vi "Log_Comando.vi"(0 "Porta":refnum<visa-resource-name>, 1 "Erro":bool, 2 "string do Comando":string, 3 "string da resposta":string, 4 "String":string, 5 "Erro de Resposta":bool, 6 "Erro Recebido":bool) -> ()   [LabVIEW 2018]
uses:
  Global_Telescopio.vi
panel:
  out "before substring":string
  out "Comando":string
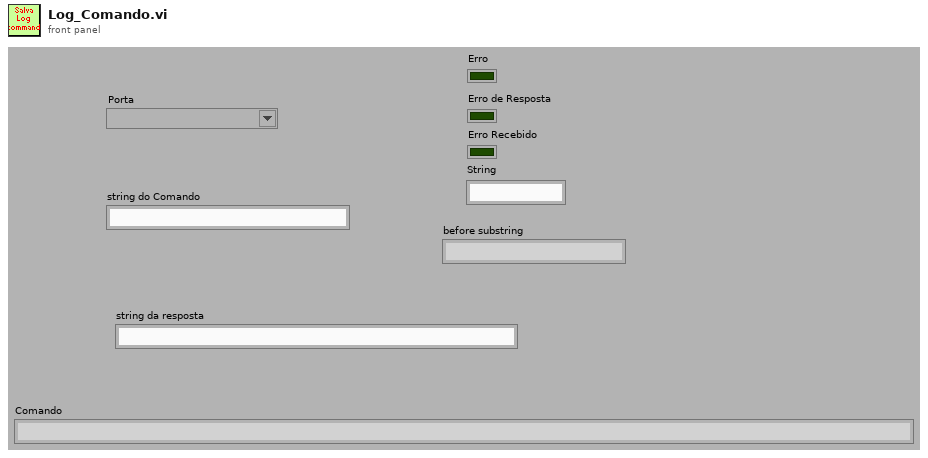
[diagram p1: front panel]
types:
  T1 = enum16{"open", "open or create", "create or replace", "create"}
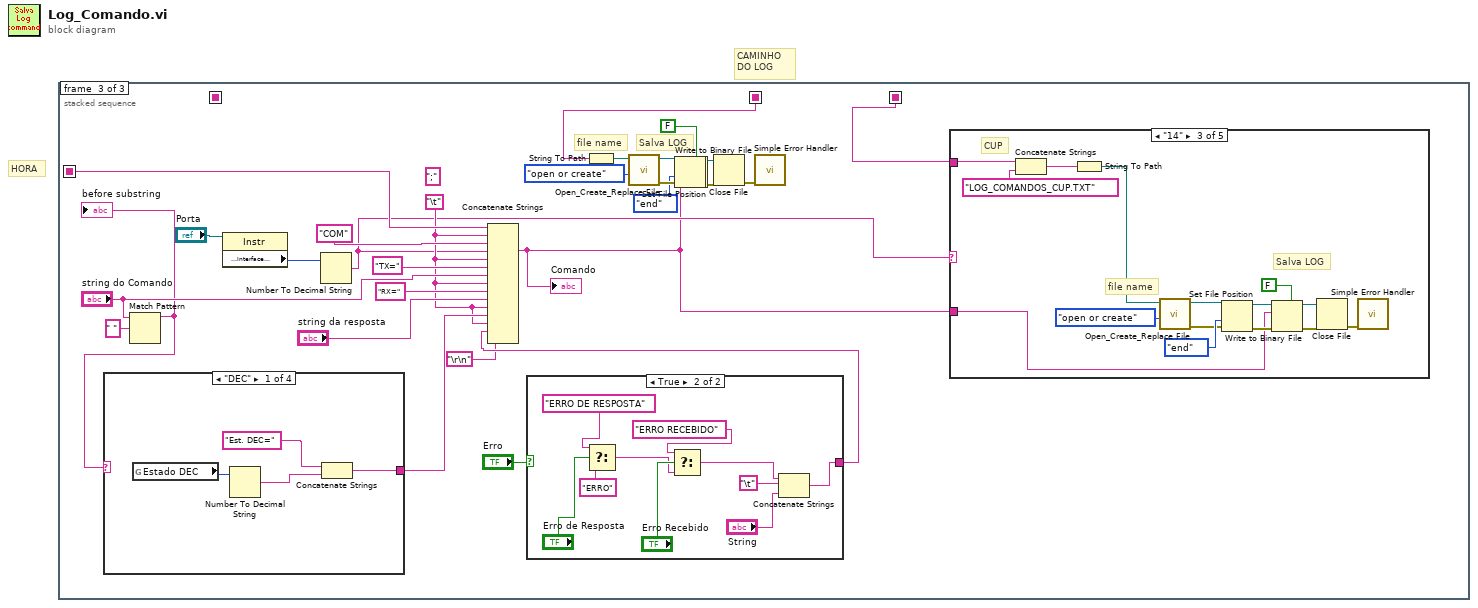
[diagram p0: block diagram]
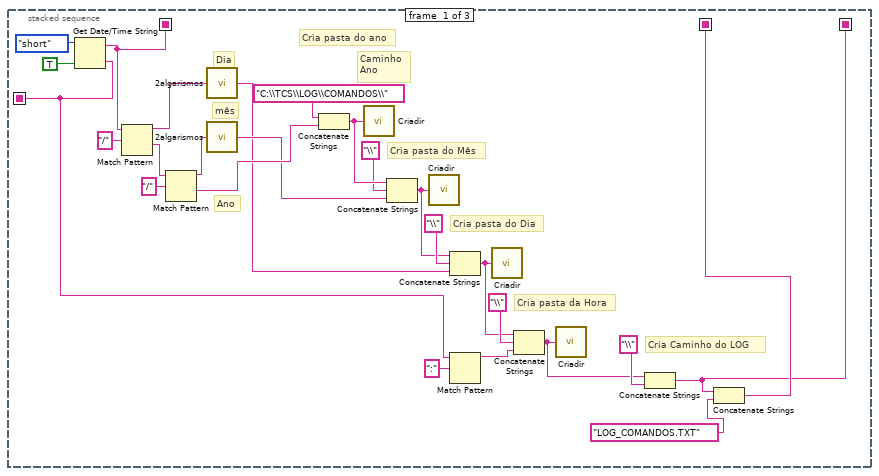
[diagram p2: hidden frame]
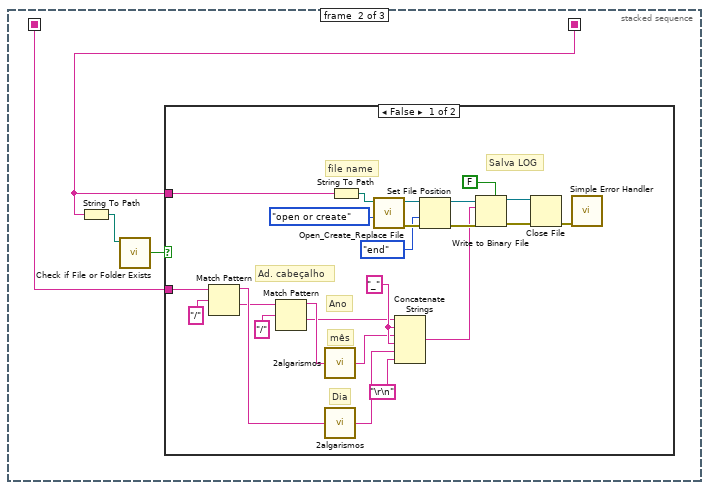
[diagram p3: hidden frame]
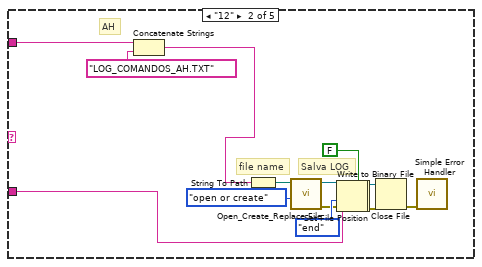
[diagram p6: hidden frame]
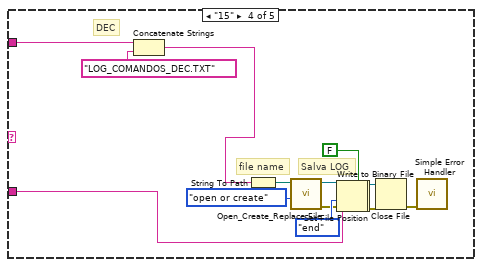
[diagram p7: hidden frame]
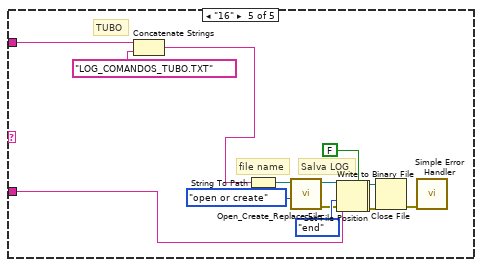
[diagram p8: hidden frame]
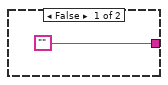
[diagram p9: hidden frame]
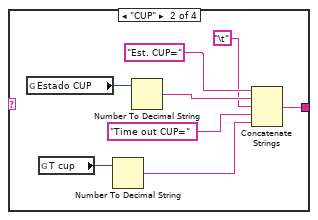
[diagram p10: hidden frame]
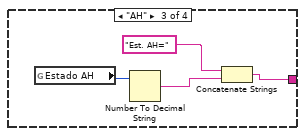
[diagram p11: hidden frame]
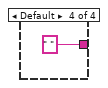
[diagram p12: hidden frame]
diagram:
  # "HORA"
  # "CAMINHO\nDO LOG"
  n1 = stacked-sequence {
    seq-local: [w2 _ _] -> [_ w29 w57]
    seq-local: [w7 _ _] -> [_ _ w81]
    seq-local: [w4 _ _] -> [_ w30 _]
    seq-local: [w1 _ _] -> [_ _ w55]
    frame #0 {
      # "Cria pasta da Hora"
      # "Cria Caminho do LOG"
      # "Cria pasta do Dia"
      # "Cria pasta do Mês"
      # "Caminho\nAno"
      # "Ano"
      # "mês"
      # "Dia"
      # "Cria pasta do ano"
      n2 = Get Date/Time String(date format (0)=enum16{"short", "long", "abbreviated"}."short", want seconds? (F)=TRUE) -> (date string=w4:string, time string=w7:string)  [unwired: 1 in]
      n3 = Match Pattern(string=w4, regular expression="/") -> (before substring=w23:string, after substring=w24:string)  [unwired: 1 in, 2 out]
      n4 = Match Pattern(string=w24, regular expression="/") -> (before substring=w22:string, after substring=w20:string)  [unwired: 1 in, 2 out]
      n5 = call "2algarismos.vi"("entrada"=w23) -> ("saida"=w14:string)
      n6 = call "2algarismos.vi"("entrada"=w22) -> ("saida"=w17:string)
      n7 = Concatenate Strings("C:\\TCS\\LOG\\COMANDOS\\" ("SOMENTE DIRETORIO"), w20) -> (w19:string)
      n8 = call "Criadir.vi"("SOMENTE DIRETORIO"=w19) -> ()  [unwired: 2 out]
      n9 = Concatenate Strings(w19, "\\" ("regular expression"), w17) -> (w15:string)
      n10 = call "Criadir.vi"("SOMENTE DIRETORIO"=w15) -> ()  [unwired: 2 out]
      n11 = Concatenate Strings(w15, "\\" ("regular expression"), w14) -> (w9:string)
      n12 = Match Pattern(string=w7, regular expression=":") -> (before substring=w6:string)  [unwired: 1 in, 3 out]
      n13 = call "Criadir.vi"("SOMENTE DIRETORIO"=w9) -> ()  [unwired: 2 out]
      n14 = Concatenate Strings(w9, "\\" ("regular expression"), w6) -> (w5:string)
      n15 = call "Criadir.vi"("SOMENTE DIRETORIO"=w5) -> ()  [unwired: 2 out]
      n16 = Concatenate Strings(w5, "\\" ("regular expression")) -> (w1:string)
      n17 = Concatenate Strings(w1, "LOG_COMANDOS.TXT" ("regular expression")) -> (w2:string)
    }
    frame #1 {
      n18 = String To Path(string=w29) -> (path=w28:path)
      n19 = call <vilib>:"Check if File or Folder Exists.vi"("path"=w28) -> ("file or folder exists?"=w27:bool)  [unwired: 8 in, 2 out]
      n20 = case shown="False" w27 {
        tunnel: w29 -> [w43 _]
        tunnel: w30 -> [w33 _]
        frame False {
          w41 = "_"
          # "Ad. cabeçalho"
          # "Ano"
          # "mês"
          # "Dia"
          # "Salva LOG"
          # "file name"
          n21 = Match Pattern(string=w33, regular expression="/") -> (before substring=w42:string, after substring=w39:string)  [unwired: 1 in, 2 out]
          n22 = Match Pattern(string=w39, regular expression="/") -> (before substring=w38:string, after substring=w37:string)  [unwired: 1 in, 2 out]
          n23 = call "2algarismos.vi"("entrada"=w38) -> ("saida"=w36:string)
          n24 = call "2algarismos.vi"("entrada"=w42) -> ("saida"=w35:string)
          n25 = String To Path(string=w43) -> (path=w47:path)
          n26 = call <vilib>:"Open_Create_Replace File.vi"("function (open:0)"=T1."open or create", "file path"=w47) -> ("error out"=w50:errorcluster, "refnum"=w53:refnum<file>)  [unwired: 6 in, 2 out]
          n27 = Concatenate Strings(w37, w41, w36, w41, w35, "\r\n") -> (w34:string)
          n28 = Set File Position(refnum=w53, from (0:start)=enum16{"start", "end", "current"}."end" ("pos mode (0:2)"), error in=w50) -> (refnum out=w46:refnum<file>, error out=w45:errorcluster)  [unwired: 1 in]
          n29 = Write to Binary File(file (use dialog)=w46, data=w34, error in=w45, 5:FALSE ("prepend array or string size? (T)")) -> (refnum out=w52:refnum<file>, error out=w51:errorcluster)  [unwired: 2 in, 1 out]
          n30 = Close File(refnum=w52, error in=w51) -> (error out=w54:errorcluster)  [unwired: 1 out]
          n31 = call <vilib>:"Simple Error Handler.vi"("error in (no error)"=w54) -> ()  [unwired: 4 in, 5 out]
        }
        frame True {
        }
      }
    }
    frame #2 {
      w61 = "\t"
      (unwired) ";"
      # "Salva LOG"
      # "file name"
      n32 = Match Pattern(string="string do Comando", regular expression=" ") -> (before substring=w64:string)  [unwired: 1 in, 3 out]
      "before substring" <- w64
      n33 = case shown="\"DEC\"" w64 {
        tunnel: [w156 w160 w168 " "] -> w63
        frame "DEC" {
          n34 = global read "Global_Telescopio.vi" "Estado DEC"() -> (w159:i32)
          n35 = Number To Decimal String(number=w159) -> (decimal integer string=w157:string)  [unwired: 1 in]
          n36 = Concatenate Strings("Est. DEC=", w157) -> (w156:string)
        }
        frame "CUP" {
          n37 = global read "Global_Telescopio.vi" "Estado CUP"() -> (w165:i32)
          n38 = global read "Global_Telescopio.vi" "T cup"() -> (w163:u32)
          n39 = Number To Decimal String(number=w163) -> (decimal integer string=w161:string)  [unwired: 1 in]
          n40 = Number To Decimal String(number=w165) -> (decimal integer string=w166:string)  [unwired: 1 in]
          n41 = Concatenate Strings("Est. CUP=", w166, "\t", "Time out CUP=", w161) -> (w160:string)
        }
        frame "AH" {
          n42 = global read "Global_Telescopio.vi" "Estado AH"() -> (w171:i32)
          n43 = Number To Decimal String(number=w171) -> (decimal integer string=w169:string)  [unwired: 1 in]
          n44 = Concatenate Strings("Est. AH=", w169) -> (w168:string)
        }
        frame Default {
        }
      }
      n45 = property class="Instr"(reference="Porta") -> ("Interface Information:Interface Number"=w83:u16)  [unwired: 1 in, 2 out]
      n46 = Number To Decimal String(number=w83) -> (decimal integer string=w58:string)  [unwired: 1 in]
      n47 = case shown="True" "Erro" {
        tunnel: ["" w146] -> w60
        frame False {
        }
        frame True {
          n48 = Select(t="ERRO DE RESPOSTA", s="Erro de Resposta", f="ERRO") -> (s? t:f=w151:string)
          n49 = Select(t="ERRO RECEBIDO", s="Erro Recebido", f=w151) -> (s? t:f=w149:string)
          n50 = Concatenate Strings(w149, "\t", "String") -> (w146:string)
        }
      }
      n51 = Concatenate Strings(w81, w61, "COM", w58, w61, "TX=", "string do Comando", w61, "RX=", "string da resposta", w61, w63, w61, w60, "\r\n") -> (w56:string)
      "Comando" <- w56
      n52 = String To Path(string=w57) -> (path=w73:path)
      n53 = call <vilib>:"Open_Create_Replace File.vi"("function (open:0)"=T1."open or create", "file path"=w73) -> ("error out"=w76:errorcluster, "refnum"=w79:refnum<file>)  [unwired: 6 in, 2 out]
      n54 = Set File Position(refnum=w79, from (0:start)=enum16{"start", "end", "current"}."end" ("pos mode (0:2)"), error in=w76) -> (refnum out=w69:refnum<file>, error out=w68:errorcluster)  [unwired: 1 in]
      n55 = Write to Binary File(file (use dialog)=w69, data=w56, error in=w68, 5:FALSE ("prepend array or string size? (T)")) -> (refnum out=w78:refnum<file>, error out=w77:errorcluster)  [unwired: 2 in, 1 out]
      n56 = Close File(refnum=w78, error in=w77) -> (error out=w80:errorcluster)  [unwired: 1 out]
      n57 = call <vilib>:"Simple Error Handler.vi"("error in (no error)"=w80) -> ()  [unwired: 4 in, 5 out]
      n58 = case shown="\"14\"" w58 {
        tunnel: w55 -> [_ w99 w114 w129 w144]
        tunnel: w56 -> [_ w85 w100 w115 w130]
        frame "False", Default {
        }
        frame "12" {
          # "Salva LOG"
          # "file name"
          # "AH"
          n59 = Concatenate Strings(w99, "LOG_COMANDOS_AH.TXT" ("regular expression")) -> (w86:string)
          n60 = String To Path(string=w86) -> (path=w94:path)
          n61 = call <vilib>:"Open_Create_Replace File.vi"("function (open:0)"=T1."open or create", "file path"=w94) -> ("error out"=w91:errorcluster, "refnum"=w88:refnum<file>)  [unwired: 6 in, 2 out]
          n62 = Set File Position(refnum=w88, from (0:start)=enum16{"start", "end", "current"}."end" ("pos mode (0:2)"), error in=w91) -> (refnum out=w95:refnum<file>, error out=w96:errorcluster)  [unwired: 1 in]
          n63 = Write to Binary File(file (use dialog)=w95, data=w85, error in=w96, 5:FALSE ("prepend array or string size? (T)")) -> (refnum out=w89:refnum<file>, error out=w90:errorcluster)  [unwired: 2 in, 1 out]
          n64 = Close File(refnum=w89, error in=w90) -> (error out=w87:errorcluster)  [unwired: 1 out]
          n65 = call <vilib>:"Simple Error Handler.vi"("error in (no error)"=w87) -> ()  [unwired: 4 in, 5 out]
        }
        frame "14" {
          # "Salva LOG"
          # "file name"
          # "CUP"
          n66 = Concatenate Strings(w114, "LOG_COMANDOS_CUP.TXT" ("regular expression")) -> (w101:string)
          n67 = String To Path(string=w101) -> (path=w109:path)
          n68 = call <vilib>:"Open_Create_Replace File.vi"("function (open:0)"=T1."open or create", "file path"=w109) -> ("error out"=w106:errorcluster, "refnum"=w103:refnum<file>)  [unwired: 6 in, 2 out]
          n69 = Set File Position(refnum=w103, from (0:start)=enum16{"start", "end", "current"}."end" ("pos mode (0:2)"), error in=w106) -> (refnum out=w110:refnum<file>, error out=w111:errorcluster)  [unwired: 1 in]
          n70 = Write to Binary File(file (use dialog)=w110, data=w100, error in=w111, 5:FALSE ("prepend array or string size? (T)")) -> (refnum out=w104:refnum<file>, error out=w105:errorcluster)  [unwired: 2 in, 1 out]
          n71 = Close File(refnum=w104, error in=w105) -> (error out=w102:errorcluster)  [unwired: 1 out]
          n72 = call <vilib>:"Simple Error Handler.vi"("error in (no error)"=w102) -> ()  [unwired: 4 in, 5 out]
        }
        frame "15" {
          # "DEC"
          # "Salva LOG"
          # "file name"
          n73 = Concatenate Strings(w129, "LOG_COMANDOS_DEC.TXT" ("regular expression")) -> (w116:string)
          n74 = String To Path(string=w116) -> (path=w124:path)
          n75 = call <vilib>:"Open_Create_Replace File.vi"("function (open:0)"=T1."open or create", "file path"=w124) -> ("error out"=w121:errorcluster, "refnum"=w118:refnum<file>)  [unwired: 6 in, 2 out]
          n76 = Set File Position(refnum=w118, from (0:start)=enum16{"start", "end", "current"}."end" ("pos mode (0:2)"), error in=w121) -> (refnum out=w125:refnum<file>, error out=w126:errorcluster)  [unwired: 1 in]
          n77 = Write to Binary File(file (use dialog)=w125, data=w115, error in=w126, 5:FALSE ("prepend array or string size? (T)")) -> (refnum out=w119:refnum<file>, error out=w120:errorcluster)  [unwired: 2 in, 1 out]
          n78 = Close File(refnum=w119, error in=w120) -> (error out=w117:errorcluster)  [unwired: 1 out]
          n79 = call <vilib>:"Simple Error Handler.vi"("error in (no error)"=w117) -> ()  [unwired: 4 in, 5 out]
        }
        frame "16" {
          # "TUBO"
          # "Salva LOG"
          # "file name"
          n80 = Concatenate Strings(w144, "LOG_COMANDOS_TUBO.TXT" ("regular expression")) -> (w131:string)
          n81 = String To Path(string=w131) -> (path=w139:path)
          n82 = call <vilib>:"Open_Create_Replace File.vi"("function (open:0)"=T1."open or create", "file path"=w139) -> ("error out"=w136:errorcluster, "refnum"=w133:refnum<file>)  [unwired: 6 in, 2 out]
          n83 = Set File Position(refnum=w133, from (0:start)=enum16{"start", "end", "current"}."end" ("pos mode (0:2)"), error in=w136) -> (refnum out=w140:refnum<file>, error out=w141:errorcluster)  [unwired: 1 in]
          n84 = Write to Binary File(file (use dialog)=w140, data=w130, error in=w141, 5:FALSE ("prepend array or string size? (T)")) -> (refnum out=w134:refnum<file>, error out=w135:errorcluster)  [unwired: 2 in, 1 out]
          n85 = Close File(refnum=w134, error in=w135) -> (error out=w132:errorcluster)  [unwired: 1 out]
          n86 = call <vilib>:"Simple Error Handler.vi"("error in (no error)"=w132) -> ()  [unwired: 4 in, 5 out]
        }
      }
    }
  }
